vi "_Update Display Property.vi"(5 "MassRange# (0)":i32, 6 "PeakParam":cluster{"MinH":dbl, "MinW":i32}={"MinH"=1.0, "MinW"=4}, 7 "Current Data":T2={"Scan#"=0, "Run Time (mS)"=0, "TIC X"=[], "TIC Y"=[], "MassRange"=[], "Fixed Mass (amu)"=1.0, "Method"={"StartT(mS)"=0, "#Cycles"=0, "PauseT(uS)"=0, "ScanType"=0, "Polarity"=0, "FixedMass"=0.0, "DelayT(mS)"=0, "Active Ch"=[], "Mass Range"=[]}} {"Method"."Mass Range"."Res" items=["High/High", "Medium/Medium", "Low/Low", "High/Medium", "High/Low", "Medium/High", "Medium/Low", "Low/High", "Low/Medium"]}, 8 "Display Refnum":refnum<vi>) -> (1 "Graph Data":T1, 2 "Active":bool, 3 "Peak List":T8[](array[typedef]))   [LabVIEW 2012]
uses:
  Type/_Peak Property.ctl
  Type/_Current Data.ctl
  Type/_XML Expt.ctl
  Type/_XML Lens.ctl
  Type/_Mass Range Property.ctl
  Type/_Mass Range Parameters.ctl
  Type/_RT Res Type.ctl
  Type/_Run Module.ctl
  Configuration/_Global Configuration.vi
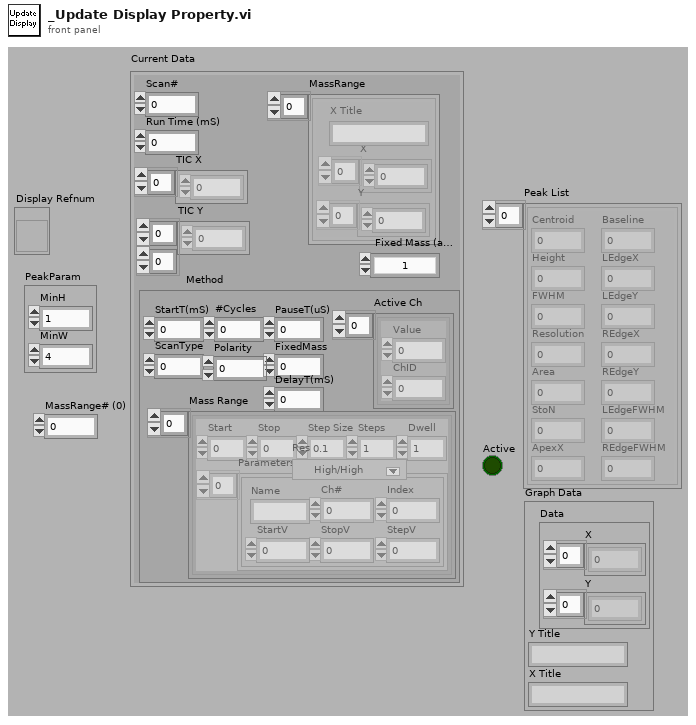
[diagram p1: front panel]
types:
  T1 = cluster{"Data":cluster{"X":dbl[], "Y":dbl[]}, "Y Title":string, "X Title":string}
  T2 = typedef "_Current Data.ctl" = cluster{"Scan#":i32, "Run Time (mS)":i32, "TIC X":dbl[], "TIC Y":dbl[][], "MassRange":cluster{"X Title":string, "X":dbl[], "Y":i32[]}[], "Fixed Mass (amu)":dbl, "Method":T3}
  T3 = typedef "_XML Expt.ctl" = cluster{"StartT(mS)":i32, "#Cycles":i32, "PauseT(uS)":i32, "ScanType":i32, "Polarity":u8, "FixedMass":dbl, "DelayT(mS)":i32, "Active Ch":T4[], "Mass Range":T5[]}
  T4 = typedef "_XML Lens.ctl" = cluster{"Value":dbl, "ChID":u8}
  T5 = typedef "_Mass Range Property.ctl" = cluster{"Start":dbl, "Stop":dbl, "Step Size":dbl, "Steps":i32, "Dwell":dbl, "Parameters":T6[], "Res":T7}
  T6 = typedef "_Mass Range Parameters.ctl" = cluster{"Name":string, "Ch#":u8, "StartV":dbl, "StopV":dbl, "StepV":dbl, "Index":u8}
  T7 = typedef "_RT Res Type.ctl" = u16
  T8 = typedef "_Peak Property.ctl" = cluster{"Centroid":dbl, "Height":dbl, "FWHM":dbl, "Resolution":dbl, "Area":dbl, "StoN":dbl, "ApexX":dbl, "Baseline":dbl, "LEdgeX":dbl, "LEdgeY":dbl, "REdgeX":dbl, "REdgeY":dbl, "LEdgeFWHM":dbl, "REdgeFWHM":dbl}
  T9 = typedef "_Run Module.ctl" = u16
  T10 = cluster{"X Title":string, "X":dbl[], "Y":i32[]}[]
  T11 = typedef "_Lens Property.ctl" = cluster{"Scan Type":u8, "Scans":i32, "Time 1":dbl, "Time 2":dbl, "Value 1":dbl, "Value 2":dbl, "Step Size":dbl}
  T12 = typedef "_Run Mode.ctl" = enum16{"MRM (Q1/Q2)", "Q1 Scan", "Q1 SRM", "Q2 Scan", "Q2 SRM", "Product Scan", "Precursor Scan", "Neutral Loss", "Neutral Gain"}
  T13 = cluster{"Lenses":T11[], "Mass Ranges":T5[], "Acquire":bool, "MCA":bool, "Q1DC EN":bool, "Q1 POL":bool, "Q3 POL":bool, "Q1 RF  EN":bool, "Averaging":bool, "Log Scale":bool, "CPS":bool, "Unit":bool, "Data Path":path, "Run Mode":T12, "Fixed Mass (amu)":dbl, "Q3DC EN":bool, "Q3 RF  EN":bool, "Negative":bool}
  T14 = cluster{cluster{"X":dbl[], "Data Out":dbl[]}, string, "X Title":string}
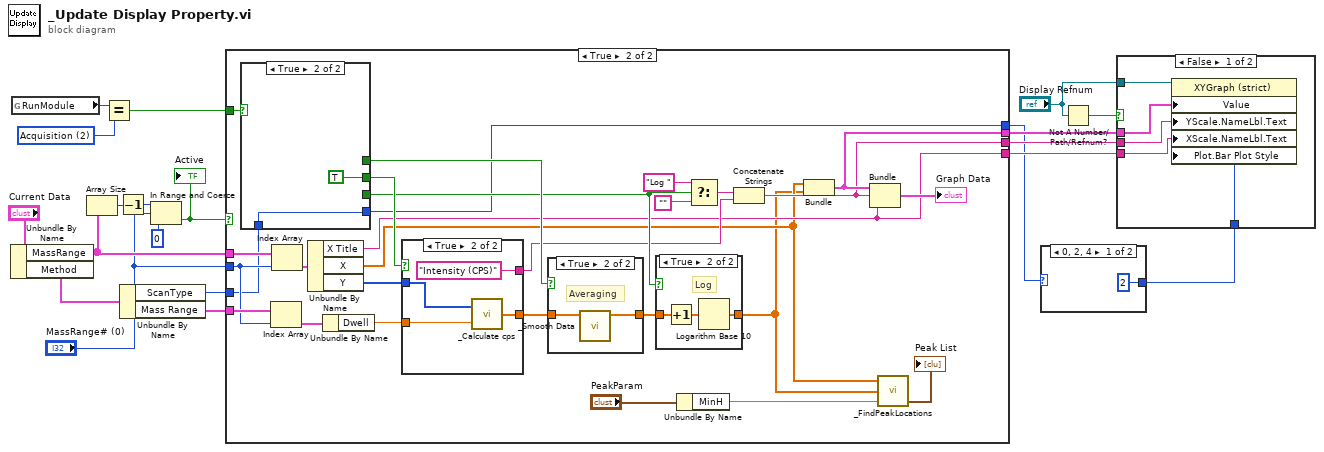
[diagram p0: block diagram]
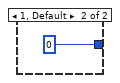
[diagram p2: hidden frame]
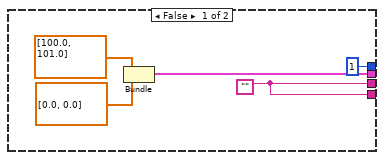
[diagram p4: hidden frame]
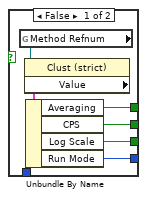
[diagram p5: hidden frame]
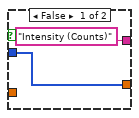
[diagram p8: hidden frame]
diagram:
  w5 = T9 2 items=["Diagnostics", "Tune", "Acquisition"] ("y")
  n1 = Unbundle By Name("Current Data") -> ("MassRange"=w18:T10, "Method"=w19:T3)
  n2 = global read "_Global Configuration.vi" "RunModule"() -> (w6:T9)
  n3 = Array Size(array=w18) -> (size(s)=w17:i32)
  n4 = Equal?(x=w6, y=w5) -> (x = y?=w4:bool)
  n5 = Decrement(x=w17) -> (x-1=w16:i32)
  n6 = Unbundle By Name(w19) -> ("ScanType"=w3:i32, "Mass Range"=w7:T5[])
  n7 = In Range and Coerce(upper limit=w16, x="MassRange# (0)", lower limit=0) -> (In Range?=w13:bool)  [unwired: 1 out]
  "Active" <- w13
  n8 = case shown="True" w13 {
    tunnel: w7 -> [_ w42]
    tunnel: w18 -> [_ w38]
    tunnel: "MassRange# (0)" -> [_ w36]
    tunnel: [w23 w35] -> w10
    tunnel: [w22 w34] -> w9
    tunnel: [w22 w33] -> w8
    tunnel: w4 -> [_ w32]
    tunnel: w3 -> [_ w31]
    tunnel: [1 ("ScanType") w30] -> w2
    frame False {
      w22 = ""
      n9 = Bundle(dbl[] [100.0, 101.0], dbl[] [0.0, 0.0]) -> (w23:cluster{dbl[], dbl[]})  [unwired: 1 out]
    }
    frame True {
      n10 = case shown="True" w32 {
        tunnel: [w57 _] -> w53
        tunnel: [w56 TRUE ("CPS")] -> w52
        tunnel: [w55 _] -> w46
        tunnel: [w54 w60] -> w30
        tunnel: w31 -> [_ w60]
        frame False {
          n11 = global read "_Global Configuration.vi" "Method Refnum"() -> (w59:refnum<vi>)
          n12 = property class="Clust (strict)"(reference=w59) -> ("Value"=w58:T13)  [unwired: 1 in, 2 out]
          n13 = Unbundle By Name(w58) -> ("Averaging"=w57:bool, "CPS"=w56:bool, "Log Scale"=w55:bool, "Run Mode"=w54:T12)
        }
        frame True {
        }
      }
      n14 = Index Array(array=w42, index=w36) -> (element=w41:T5)
      n15 = Index Array(array=w38, index=w36) -> (element=w43:cluster{"X Title":string, "X":dbl[], "Y":i32[]})
      n16 = Unbundle By Name(w43) -> ("X Title"=w33:string, "X"=w29:dbl[], "Y"=w40:i32[])
      n17 = Unbundle By Name(w41) -> ("Dwell"=w39:dbl)
      n18 = case shown="True" w52 {
        tunnel: [w69 w74] -> w51
        tunnel: ["Intensity (Counts)" "Intensity (CPS)"] -> w45
        tunnel: w40 -> [w69 w72]
        tunnel: w39 -> [_ w71]
        frame False {
        }
        frame True {
          n19 = call "_Calculate cps.vi"("Dwell (mS)"=w71, "Raw Counts"=w72) -> ("Data in cps"=w74:dbl[])
        }
      }
      n20 = case shown="True" w53 {
        tunnel: w51 -> [w66 w68]
        tunnel: [w66 w67] -> w50
        frame False {
        }
        frame True {
          # "Averaging"
          n21 = call "_Smooth Data.vi"("Data In"=w68) -> ("Data Out"=w67:dbl[])  [unwired: 6 out]
        }
      }
      n22 = case shown="True" w46 {
        tunnel: w50 -> [w62 w65]
        tunnel: [w62 w64] -> w28
        frame False {
        }
        frame True {
          # "Log"
          n23 = Increment(x=w65) -> (x+1=w63:dbl[])
          n24 = Logarithm Base 10(1:w63) -> (0:w64:dbl[])
        }
      }
      n25 = Unbundle By Name("PeakParam") -> ("MinH"=w27:dbl)
      n26 = Select(t="Log ", s=w46, f="") -> (s? t:f=w49:string)
      n27 = Concatenate Strings(w49, w45) -> (w34:string)
      n28 = Bundle("X"=w29, "Data Out"=w28) -> (w35:cluster{"X":dbl[], "Data Out":dbl[]})  [unwired: 1 out]
      n29 = Bundle(w35, w34, "X Title"=w33) -> (→"Graph Data":T14)  [unwired: 1 out]
      n30 = call "_FindPeakLocations.vi"("threshold"=w27, "Intensities"=w28, "Masses"=w29) -> ("Peak List"=→"Peak List":T8[])  [unwired: 1 in, 1 out]
    }
  }
  n31 = case shown="0, 2, 4" w2 {
    tunnel: [u8 2 ("Plot.Bar Plot Style") u8 0 ("Plot.Bar Plot Style")] -> w1
    frame 0, 2, 4 {
    }
    frame 1, Default {
    }
  }
  n32 = Not A Number/Path/Refnum?(number/path/refnum="Display Refnum") -> (NaN/Path/Refnum?=w12:bool)
  n33 = case shown="False" w12 {
    tunnel: "Display Refnum" -> [w81 _]
    tunnel: w10 -> [w80 _]
    tunnel: w9 -> [w79 _]
    tunnel: w8 -> [w78 _]
    tunnel: w1 -> [w77 _]
    frame False {
      n34 = property class="XYGraph (strict)"(reference=w81, "Value"=w80, "YScale.NameLbl.Text"=w79, "XScale.NameLbl.Text"=w78, "Plot.Bar Plot Style"=w77) -> ()  [unwired: 1 in, 2 out]
    }
    frame True {
    }
  }
